vi "Reversing_Switch.vi"(8 "error in":errorcluster, 11 "Reversing Switch Function":T1) -> (0 "error out":errorcluster, 3 "Verfied":bool)   [LabVIEW 2012]
uses:
  Reversing_Switch.ctl
panel:
  # "Reversing Switch"
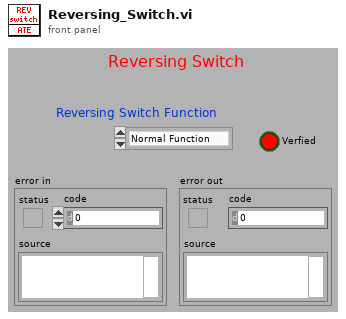
[diagram p1: front panel]
types:
  T1 = typedef "Reversing_Switch.ctl" = enum16{"Normal Function", "Reversing Function"}
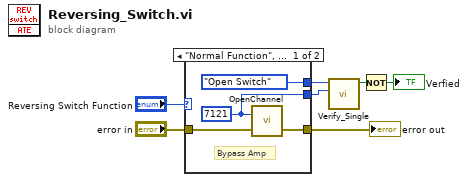
[diagram p0: block diagram]
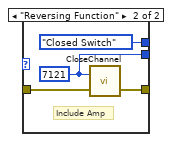
[diagram p2: hidden frame]
diagram:
  n1 = case shown="\"Normal Function\", Default" "Reversing Switch Function" {
    tunnel: "error in" -> [w11 w15]
    tunnel: [w10 w14] -> w5
    tunnel: [w9 w13] -> w4
    tunnel: [enum16{"Open Switch", "Closed Switch"}."Open Switch" ("Switch Functin") enum16{"Open Switch", "Closed Switch"}."Closed Switch" ("Switch Functin")] -> w3
    frame "Normal Function", Default {
      w9 = 7121
      # "Bypass Amp"
      n2 = call "OpenChannel.vi"("error in (no error)"=w11, "Channel ID"=w9) -> ("error out"=w10:errorcluster)  [unwired: 1 in]
    }
    frame "Reversing Function" {
      w13 = 7121
      # "Include Amp"
      n3 = call "CloseChannel.vi"("error in (no error)"=w15, "Channel ID"=w13) -> ("error out"=w14:errorcluster)  [unwired: 1 in]
    }
  }
  "error out" <- w5
  n4 = call "Verify_Single.vi"("Switch ID"=w4, "Switch Functin"=w3) -> ("Verfied"=w2:bool)  [unwired: 8 in, 1 out]
  n5 = Not(x=w2) -> (.not. x?=→"Verfied":bool)
